vi "niRFUtil RFHS Benchmark Register.vi"(0 "Special ID":string, 5 "Owner":u32) -> (4 "ID":u32)   [LabVIEW 2015, in "niRFUtil.lvlib"]
uses:
  niRFUtil.lvlib
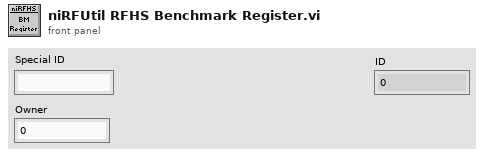
[diagram p1: front panel]
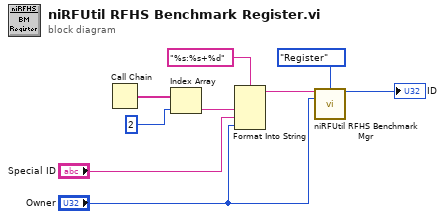
[diagram p0: block diagram]
diagram:
  n1 = Call Chain() -> (call chain=w9:string[])
  n2 = Index Array(array=w9, index=2) -> (element=w5:string)
  n3 = Format Into String(format string="%s:%s+%d", w5, "Special ID", "Owner") -> (resulting string=w2:string)  [unwired: 2 in, 1 out]
  n4 = call "niRFUtil RFHS Benchmark Mgr.vi"("String"=w2, "What"=enum16{"Register"}."Register", "Owner"="Owner") -> ("ID"=→"ID":u32)  [unwired: 11 in, 1 out]
